vi "Generate_Clear_Errors.vi"(8 "error in (no error)":errorcluster, 9 "location":T1, 11 "VI in":refnum<vi>) -> (0 "error out":errorcluster, 1 "error out term":refnum<vi>, 2 "error in term":refnum<vi>, 3 "object refnum":refnum<vi>)   [LabVIEW 2025]
uses:
  <vilib>/Utility/miscctls.llb/LVPointTypeDef.ctl
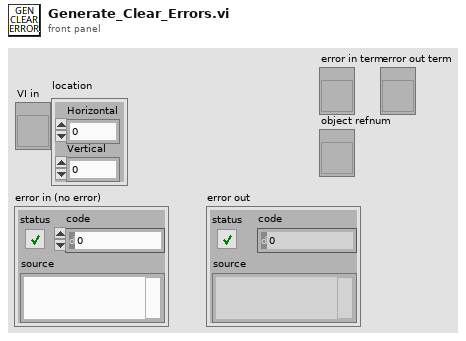
[diagram p1: front panel]
types:
  T1 = typedef "LVPointTypeDef.ctl" = cluster{"Horizontal":i16, "Vertical":i16}
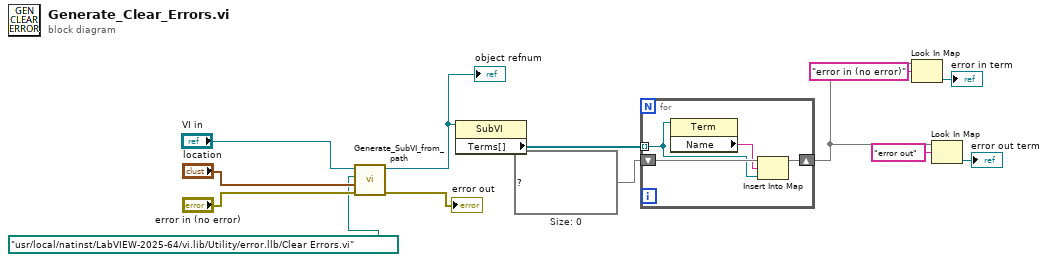
[diagram p0: block diagram]
diagram:
  w7 = map{string, refnum<vi>} {}  # Size: 0
  n1 = call "Generate_SubVI_from_path.vi"("error in (no error)"="error in (no error)", "location"="location", "path"=path "/usr/local/natinst/LabVIEW-2025-64/vi.lib/Utility/error.llb/Clear Errors.vi", "VI in"="VI in") -> ("error out"=→"error out":errorcluster, "SubVI out"=w8:refnum<vi>)  [unwired: 6 in]
  "object refnum" <- w8
  n2 = property class="SubVI"(reference=w8) -> ("Terms[]"=w6:refnum<vi>[])  [unwired: 1 in, 2 out]
  n3 = for {
    tunnel: w6 -> [w14] mode=indexing
    shift-right: [w16] -> w3
    shift-left: w7 -> [w17]
    n4 = property class="Term"(reference=w14) -> ("Name"=w15:string)  [unwired: 1 in, 2 out]
    n5 = Insert Into Map(map in=w17, key=w15, value=w14) -> (map out=w16:map{string, refnum<vi>})  [unwired: 2 out]
  }
  n6 = Look In Map(map=w3, key="error in (no error)") -> (value=→"error in term":refnum<vi>)  [unwired: 1 in, 1 out]
  n7 = Look In Map(map=w3, key="error out") -> (value=→"error out term":refnum<vi>)  [unwired: 1 in, 1 out]
